vi "K_S30_VISA CalculateCRC16.vi"(7 "msg without CRC":u8[](array[numeric])) -> (0 "CRC16":u16, 1 "CRC Lo":u8, 2 "CRC Hi":u8, 3 "msg and CRC":u8[](array[numeric]))   [LabVIEW 2012]
panel:
  # "Calculate CRC-16 checksum and append it to the message\nV1.1, b.v."
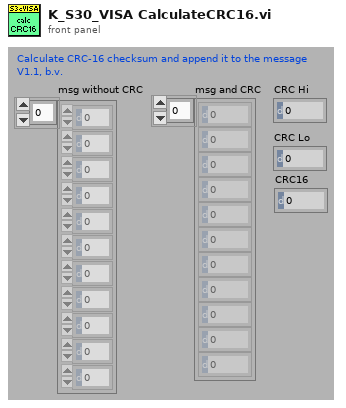
[diagram p1: front panel]
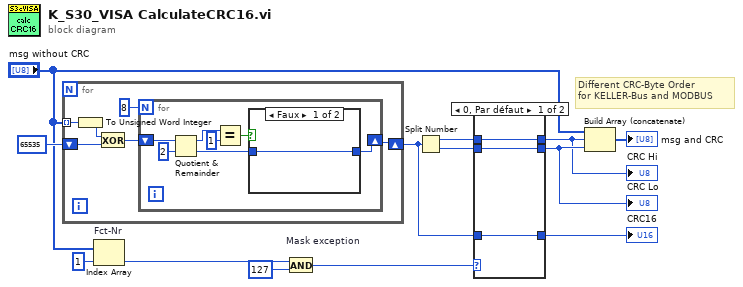
[diagram p0: block diagram]
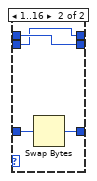
[diagram p2: hidden frame]
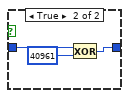
[diagram p3: hidden frame]
diagram:
  # "Different CRC-Byte Order  \nfor KELLER-Bus and MODBUS"
  n1 = for {
    tunnel: "msg without CRC" -> [w19] mode=indexing
    shift-right: [w15] -> w7
    shift-left: u16 65535 -> [w16]
    n2 = To Unsigned Word Integer(number=w19) -> (unsigned 16bit integer=w14:u16)
    n3 = Exclusive Or(1:w16, 2:w14) -> (0:w17:u16)
    n4 = for {
      N: 8 -> [_]
      shift-right: [w20] -> w15
      shift-left: w17 -> [w26]
      n5 = Quotient & Remainder(x=w26, y=u16 2) -> (x-y*floor(x/y)=w24:u16, floor(x/y)=w21:u16)
      n6 = Equal?(x=w24, y=u16 1) -> (x = y?=w22:bool)
      n7 = case shown="Faux" w22 {
        tunnel: w21 -> [w27 w30]
        tunnel: [w27 w28] -> w20
        frame False {
        }
        frame True {
          n8 = Exclusive Or(1:u16 40961, 2:w30) -> (0:w28:u16)
        }
      }
    }
  }
  n9 = Index Array "Fct-Nr"(array="msg without CRC", index=1 ("Index")) -> (element=w4:u8)
  n10 = And "Mask exception"(x=w4, y=u8 127) -> (x .and. y?=w2:u8)
  n11 = Split Number(x=w7) -> (hi(x)=w11:u8, lo(x)=w10:u8)
  n12 = case shown="0, Par défaut" w2 {
    tunnel: w11 -> [w33 w37]
    tunnel: [w33 w36] -> w8
    tunnel: [w32 w37] -> w9
    tunnel: w10 -> [w32 w36]
    tunnel: w7 -> [w31 w35]
    tunnel: [w31 w34] -> w6
    frame 0, Default {
    }
    frame 1..16 {
      n13 = Swap Bytes(anything=w35) -> (byte swapped=w34:u16)
    }
  }
  "CRC Hi" <- w8
  "CRC Lo" <- w9
  "CRC16" <- w6
  n14 = Build Array (concatenate)("msg without CRC", w8, w9) -> (→"msg and CRC":u8[])
